vi "缺口位置.vi"(8 "是否缺口判断标准":cluster{dbl, dbl}, 9 "圆心到分界点半径":sgl[](array[numeric]), 10 "分界点坐标":cluster{dbl, dbl}[](array[cluster]), 11 "Img输入":T1) -> (0 "缺口数量":i32, 2 "存储缺口中心位置":cluster{"X":sgl, "Y":sgl}[](array[cluster]), 4 "每个缺口像素点数量":i32[](array[numeric]))   [LabVIEW 2014]
uses:
  <vilib>/vision/Image Controls.llb/IMAQ Image.ctl
panel:
  out "记录连续多少个像素不是缺口":i32
  out "记录连续多少个像素是缺口":i32
  out "存储当前缺口的默认位置":cluster{"X":sgl, "Y":sgl}[](array[cluster])
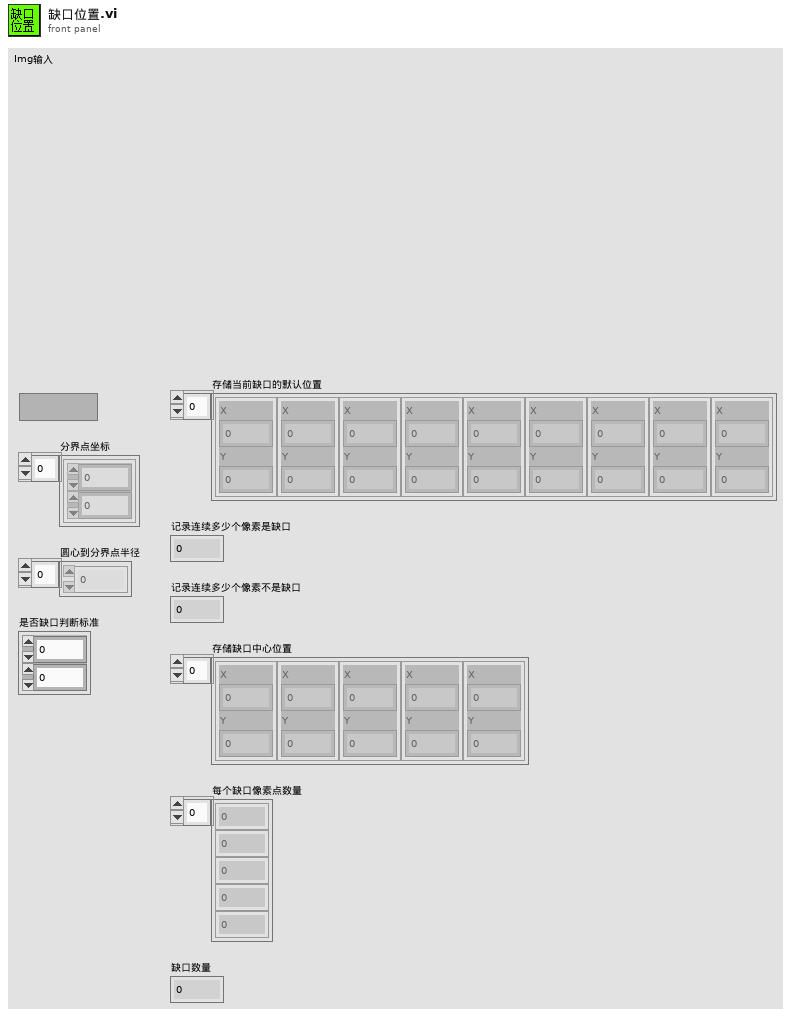
[diagram p1: front panel]
types:
  T1 = typedef "IMAQ Image.ctl" = refnum<image>
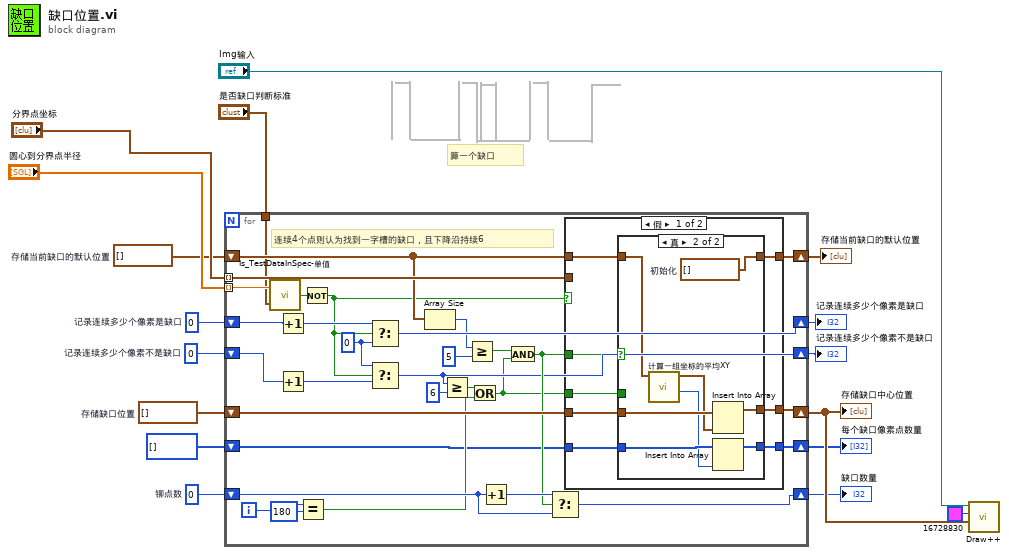
[diagram p0: block diagram]
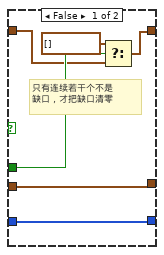
[diagram p2: hidden frame]
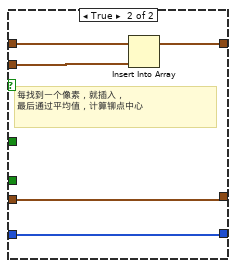
[diagram p3: hidden frame]
diagram:
  w7 = 0  # 记录连续多少个像素不是缺口
  w4 = cluster{"X":sgl, "Y":sgl}[] []  # 存储缺口位置
  w3 = cluster{"X":sgl, "Y":sgl}[] []  # 存储当前缺口的默认位置
  w2 = 0  # 记录连续多少个像素是缺口
  w1 = 0  # 铆点数
  # "算一个缺口"
  n1 = for {
    tunnel: "圆心到分界点半径" -> [w19] mode=indexing
    shift-right: [w47] -> w9
    shift-left: w1 -> [w46]
    shift-right: [w35] -> w12
    shift-left: w2 -> [w37]
    tunnel: "分界点坐标" -> [w45] mode=indexing
    shift-right: [w44] -> w8
    shift-left: w3 -> [w28]
    shift-right: [w42] -> w15
    shift-left: w4 -> [w43]
    shift-right: [w25] -> w13
    shift-left: w7 -> [w34]
    shift-right: [w24] -> w11
    shift-left: i32[] [] -> [w23]
    tunnel: "是否缺口判断标准" -> [w18]
    i -> [w38]
    w32 = 0 ("f")
    # "连续4个点则认为找到一字槽的缺口，且下降沿持续6"
    n2 = call "Is_TestDataInSpec-单值.vi"("量测规格"=w18, "相机量测结果"=w19) -> ("在规格内"=w20:bool)
    n3 = Increment(x=w37) -> (x+1=w36:i32)
    n4 = Increment(x=w34) -> (x+1=w33:i32)
    n5 = Equal?(x=w38, y=180) -> (x = y?=w39:bool)
    n6 = Not(x=w20) -> (.not. x?=w21:bool)
    n7 = Select(t=w36, s=w21, f=w32) -> (s? t:f=w35:i32)
    n8 = Select(t=w32, s=w21, f=w33) -> (s? t:f=w25:i32)
    n9 = Array Size(array=w28) -> (size(s)=w27:i32)
    n10 = Greater Or Equal?(x=w25, y=6) -> (x >= y?=w30:bool)
    n11 = Greater Or Equal?(x=w27, y=5) -> (x >= y?=w29:bool)
    n12 = Or(x=w30, y=w39) -> (x .or. y?=w22:bool)
    n13 = Increment(x=w46) -> (x+1=w48:i32)
    n14 = And(x=w29, y=w22) -> (x .and. y?=w41:bool)
    n15 = Select(t=w48, s=w41, f=w46) -> (s? t:f=w47:i32)
    n16 = case shown="假" w21 {
      tunnel: w28 -> [w52 w75]
      tunnel: w45 -> [_ w74]
      tunnel: [w53 w73] -> w44
      tunnel: w43 -> [w56 w72]
      tunnel: w41 -> [w54 _]
      tunnel: [w55 w72] -> w42
      tunnel: [w51 w71] -> w24
      tunnel: w23 -> [w50 w71]
      tunnel: w22 -> [w49 _]
      frame False {
        n17 = case shown="真" w54 {
          tunnel: w56 -> [w62 w70]
          tunnel: [w62 w68] -> w55
          tunnel: [w58 w67] -> w53
          tunnel: w52 -> [w59 w63]
          tunnel: [w61 w66] -> w51
          tunnel: w50 -> [w61 w65]
          tunnel: w49 -> [w60 _]
          frame False {
            # "只有连续若干个不是\n缺口，才把缺口清零"
            n18 = Select(t=cluster{"X":sgl, "Y":sgl}[] [], s=w60, f=w59) -> (s? t:f=w58:cluster{"X":sgl, "Y":sgl}[])
          }
          frame True {
            w67 = cluster{"X":sgl, "Y":sgl}[] []  # 初始化
            n19 = call "计算一组坐标的平均XY.vi"("存储当前铆点的默认位置"=w63) -> ("大小"=w64:i32, "簇"=w69:cluster{"mean":dbl, "mean":dbl})  [unwired: 9 in]
            n20 = Insert Into Array(array=w70, new element=w69) -> (w68:cluster{"X":sgl, "Y":sgl}[])  [unwired: 1 in]
            n21 = Insert Into Array(array=w65, new element=w64) -> (w66:i32[])  [unwired: 1 in]
          }
        }
      }
      frame True {
        # "每找到一个像素，就插入，\n最后通过平均值，计算铆点中心"
        n22 = Insert Into Array(array=w75, new element=w74) -> (w73:cluster{"X":sgl, "Y":sgl}[])  [unwired: 1 in]
      }
    }
  }
  "缺口数量" <- w9
  "存储缺口中心位置" <- w15
  "存储当前缺口的默认位置" <- w8
  "每个缺口像素点数量" <- w11
  "记录连续多少个像素是缺口" <- w12
  "记录连续多少个像素不是缺口" <- w13
  n23 = call "Draw++.vi"("PosArray"=w15, "Color"=u32 16728830, "Image In"="Img输入") -> ()  [unwired: 1 in, 1 out]
